vi "myRIO_main.vi"   [LabVIEW 2013]
uses:
  My Computer/Controls/Sepios_status.ctl
  <vilib>/myRIO/Common/Instrument Driver Framework/myRIO v1.0/UART/vis/myRIO v1.0 Close UART.vi
  <vilib>/myRIO/Common/Instrument Driver Framework/Utilities/vis/FPGA Ref Manager.vi
  <vilib>/myRIO/Common/Instrument Driver Framework/myRIO v1.0/myRIO v1.0 Reset FPGA.vi
  <vilib>/myRIO/Instrument Drivers/Utilities/Utilities.lvlib
types:
  T1 = enum16{"Run", "Standby", "ErrorHandler", "Debug"}
  T2 = typedef "Sepios_status.ctl" = enum16{"Standby", "Running", "Filming", "Error"}
  T3 = cluster{"Water Density":dbl, "SB_parameters":cluster{"x0":dbl, "U_full":dbl, "U_empty":dbl}}
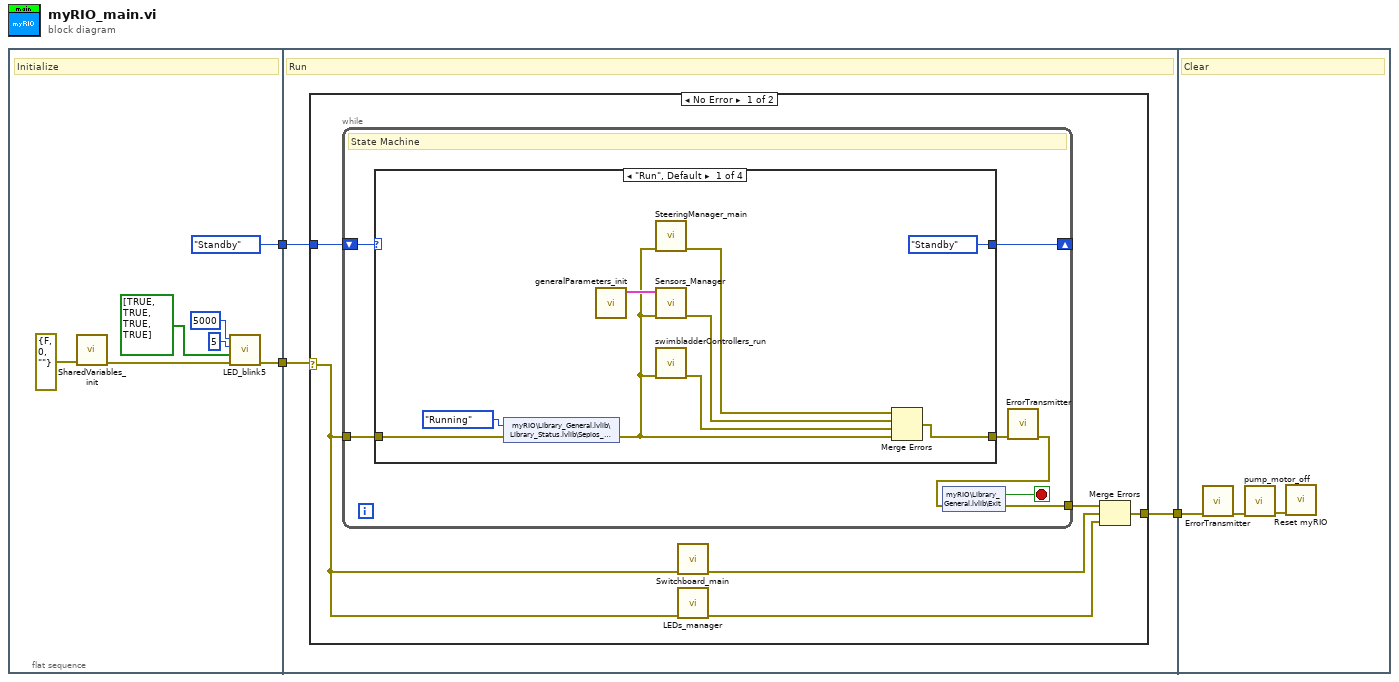
[diagram p0: block diagram]
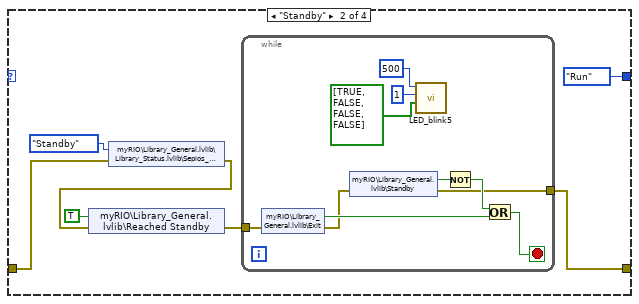
[diagram p2: hidden frame]
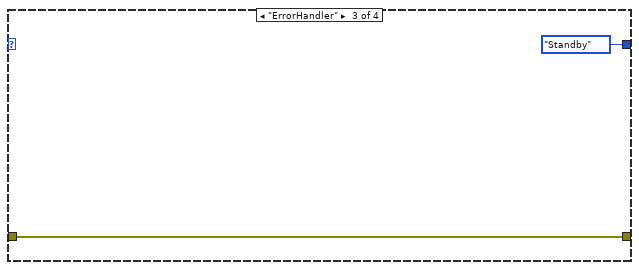
[diagram p3: hidden frame]
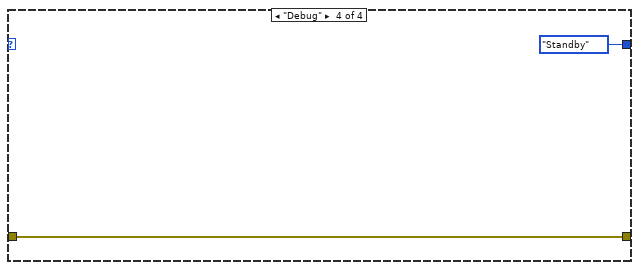
[diagram p4: hidden frame]
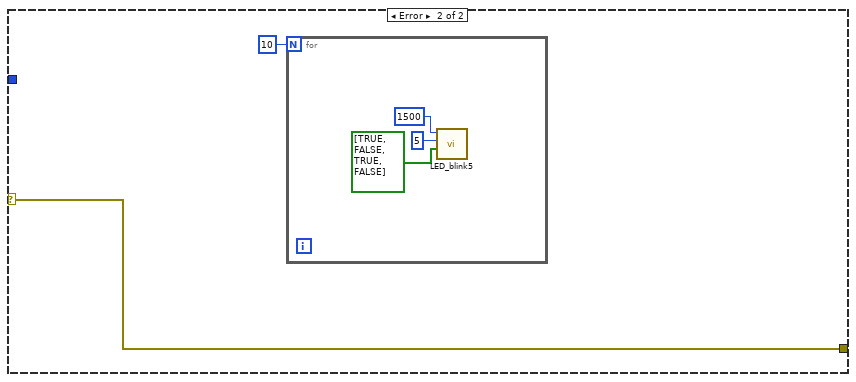
[diagram p5: hidden frame]
diagram:
  n1 = flat-sequence {
    tunnel: [T1."Standby"] -> w3
    tunnel: [w7] -> w1
    tunnel: w3 -> [w13]
    tunnel: [w12] -> w2
    tunnel: w1 -> [w11]
    tunnel: w2 -> [w64]
    frame #0 {
      # "Initialize"
      n2 = call "SharedVariables_init.vi"("error in (no error)"=errorcluster {"status"=FALSE, "code"=0, "source"=""}) -> ("error out"=w8:errorcluster)  [unwired: 10 in]
      n3 = call "LED_blink5.vi"("Error In"=w8, "LEDs"=bool[] [TRUE, TRUE, TRUE, TRUE], "Amount"=u32 5, "Time (ms)"=u32 5000) -> ("Error Out"=w7:errorcluster)  [unwired: 7 in]
    }
    frame #1 {
      # "Run"
      n4 = case shown="No Error" w11 {
        selector: w11 -> [w14 w57]
        tunnel: w13 -> [w19 _]
        tunnel: [w17 w57] -> w12
        frame No Error {
          n5 = while {
            shift-right: [w23] -> _
            shift-left: w19 -> [w26]
            tunnel: w14 -> [w25]
            tunnel: [w21] -> w18
            stop <- w24 stop-if-true
            # "State Machine"
            n6 = case shown="\"Run\", Default" w26 {
              tunnel: w25 -> [w27 w36 w54 w56]
              tunnel: [w31 w39 w54 w56] -> w22
              tunnel: [T1."Standby" T1."Run" T1."Standby" T1."Standby"] -> w23
              frame "Run", Default {
                n7 = shared-variable "myRIO\\Library_General.lvlib\\Library_Status.lvlib\\Sepios_Status"(Sepios_status."Running" ("Sepios_Status"), error in=w27) -> (error out=w28:errorcluster)
                n8 = call "generalParameters_init.vi"() -> ("General Parameters"=w30:T3)  [unwired: 11 in]
                n9 = call "SteeringManager_main.vi"("Error in"=w28) -> ("Error Out"=w32:errorcluster)  [unwired: 10 in]
                n10 = call "Sensors_Manager.vi"("error in (no error)"=w28, "Initial Settings"=w30) -> ("error out"=w33:errorcluster)  [unwired: 9 in]
                n11 = call "swimbladderControllers_run.vi"("error in (no error)"=w28) -> ("error out"=w34:errorcluster)  [unwired: 10 in]
                n12 = Merge Errors(w32, w33, w34, w28) -> (w31:errorcluster)
              }
              frame "Standby" {
                n13 = shared-variable "myRIO\\Library_General.lvlib\\Library_Status.lvlib\\Sepios_Status"(Sepios_status."Standby" ("Sepios_Status"), error in=w36) -> (error out=w37:errorcluster)
                n14 = shared-variable "myRIO\\Library_General.lvlib\\Reached Standby"(TRUE ("Reached Standby"), error in=w37) -> (error out=w40:errorcluster)
                n15 = while {
                  tunnel: w40 -> [w48]
                  tunnel: [w46] -> w39
                  stop <- w51 stop-if-true
                  n16 = shared-variable "myRIO\\Library_General.lvlib\\Exit"(error in=w48) -> (w52:bool, error out=w47:errorcluster)
                  n17 = shared-variable "myRIO\\Library_General.lvlib\\Standby"(error in=w47) -> (w50:bool, error out=w46:errorcluster)
                  n18 = call "LED_blink5.vi"("LEDs"=bool[] [TRUE, FALSE, FALSE, FALSE], "Amount"=u32 1, "Time (ms)"=u32 500) -> ()  [unwired: 8 in, 1 out]
                  n19 = Not(x=w50) -> (.not. x?=w49:bool)
                  n20 = Or(x=w49, y=w52) -> (x .or. y?=w51:bool)
                }
              }
              frame "ErrorHandler" {
              }
              frame "Debug" {
              }
            }
            n21 = call "ErrorTransmitter.vi"("Error In"=w22) -> ("Error Out"=w20:errorcluster)  [unwired: 10 in]
            n22 = shared-variable "myRIO\\Library_General.lvlib\\Exit"(error in=w20) -> (w24:bool, error out=w21:errorcluster)
          }
          n23 = call "Switchboard_main.vi"("Error In"=w14) -> ("Error Out"=w15:errorcluster)  [unwired: 10 in]
          n24 = call "LEDs_manager.vi"("Error In"=w14) -> ("Error Out"=w16:errorcluster)  [unwired: 10 in]
          n25 = Merge Errors(w18, w15, w16) -> (w17:errorcluster)
        }
        frame Error {
          n26 = for {
            N: 10 -> [_]
            n27 = call "LED_blink5.vi"("LEDs"=bool[] [TRUE, FALSE, TRUE, FALSE], "Amount"=u32 5, "Time (ms)"=u32 1500) -> ()  [unwired: 8 in, 1 out]
          }
        }
      }
    }
    frame #2 {
      # "Clear"
      n28 = call "ErrorTransmitter.vi"("Error In"=w64) -> ("Error Out"=w63:errorcluster)  [unwired: 10 in]
      n29 = call "pump_motor_off.vi"("error in (no error)"=w63) -> ("error out"=w62:errorcluster)  [unwired: 10 in]
      n30 = call <vilib>:"Reset myRIO.vi"("error in (no error)"=w62) -> ()  [unwired: 10 in, 1 out]
    }
  }
